vi "GetResult.vi"(2 "ReadBuff":string) -> (4 "Error?":bool, 6 "Addr":u8, 7 "Cmd":u8, 8 "Data":u8)   [LabVIEW 2012, in "DevControl.lvclass"]
uses:
  DevControl.lvclass
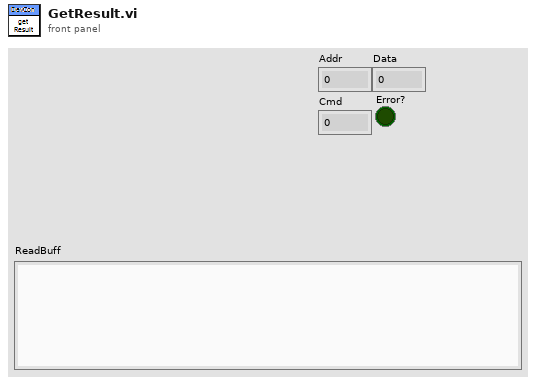
[diagram p1: front panel]
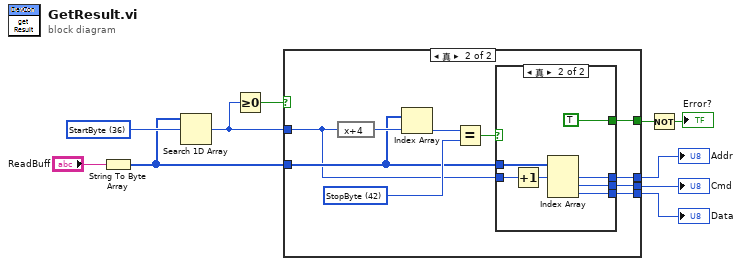
[diagram p0: block diagram]
diagram:
  w9 = u8 36 items=["StopByte"=42, "StartByte"=36] ("FunByte")
  n1 = String To Byte Array(string="ReadBuff") -> (unsigned byte array=w6:u8[])
  n2 = Search 1D Array(1D array=w6, element=w9) -> (index of element=w7:i32)  [unwired: 1 in]
  n3 = Greater Or Equal To 0?(x=w7) -> (x >= 0?=w8:bool)
  n4 = case shown="真" w8 {
    tunnel: w7 -> [_ w16]
    tunnel: w6 -> [_ w17]
    tunnel: [_ w14] -> w5
    tunnel: [_ w13] -> w4
    tunnel: [_ w12] -> w3
    tunnel: [_ w11] -> w2
    frame False {
    }
    frame True {
      w18 = u8 42 items=["StopByte"=42, "StartByte"=36] ("FunByte")
      n5 = expression code="x+4"(w16) -> (w20:i32)
      n6 = Index Array(array=w17, index=w20) -> (element=w19:u8)
      n7 = Equal?(x=w19, y=w18) -> (x = y?=w15:bool)
      n8 = case shown="真" w15 {
        tunnel: w17 -> [_ w27]
        tunnel: w16 -> [_ w25]
        tunnel: [_ w24] -> w14
        tunnel: [_ w23] -> w13
        tunnel: [_ w22] -> w12
        tunnel: [_ TRUE] -> w11
        frame False {
        }
        frame True {
          n9 = Increment(x=w25) -> (x+1=w26:i32)
          n10 = Index Array(array=w27, index #1=w26) -> (element #1=w24:u8, element #2=w23:u8, element #3=w22:u8)  [unwired: 2 in]
        }
      }
    }
  }
  "Addr" <- w5
  "Cmd" <- w4
  "Data" <- w3
  n11 = Not(x=w2) -> (.not. x?=→"Error?":bool)
